vi "Get_InteropAssembly_Data.vi"(8 "error in (no error)":errorcluster, 11 "Class in":refnum<class "AB_InteropAssembly.lvclass">) -> (0 "error out":errorcluster, 2 "data":T1, 3 "Class out":refnum<class "AB_InteropAssembly.lvclass">)   [LabVIEW 2020, in "AB_InteropAssembly.lvclass"]
uses:
  <vilib>/AppBuilder/AB_Classes/InteropAssembly/AB_InteropAssembly.lvclass
  <vilib>/AppBuilder/AB_Classes/InteropAssembly/AB_InteropAssembly.ctl
  <vilib>/AppBuilder/AB_Classes/InteropAssembly/AB_InteropAssembly.lvclass/AB_InteropAssembly.ctl
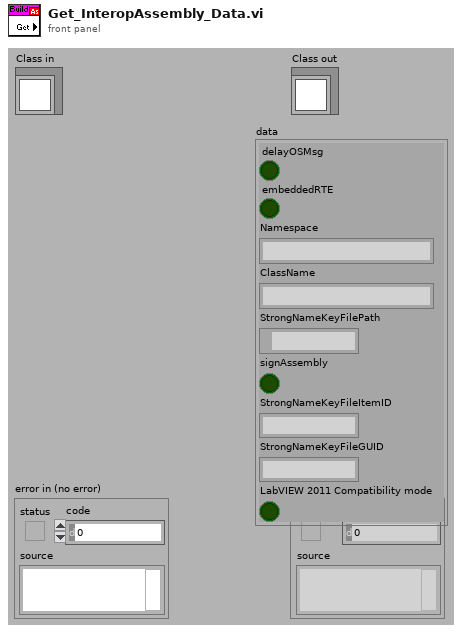
[diagram p1: front panel]
types:
  T1 = typedef "AB_InteropAssembly.ctl" = cluster{"delayOSMsg":bool, "embeddedRTE":bool, "Namespace":string, "ClassName":string, "StrongNameKeyFilePath":path, "signAssembly":bool, "StrongNameKeyFileItemID":string, "StrongNameKeyFileGUID":string, "LabVIEW 2011 Compatibility mode":bool}
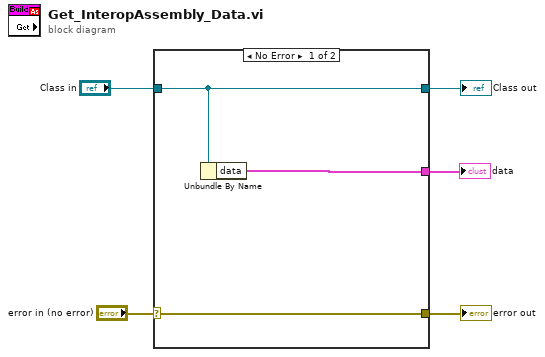
[diagram p0: block diagram]
diagram:
  n1 = case shown="No Error" "error in (no error)" {
    selector: "error in (no error)" -> [w8 w10]
    tunnel: [w8 w10] -> w4
    tunnel: [w7 w9] -> w2
    tunnel: "Class in" -> [w7 w9]
    tunnel: [w6 _] -> w1
    frame No Error {
      n2 = Unbundle By Name(w7) -> ("data"=w6:T1)
    }
    frame Error {
    }
  }
  "error out" <- w4
  "Class out" <- w2
  "data" <- w1
